vi "CRYGet Heterodyne Curve.vi"(9 "Unit Info In":T5={"Y unit In"="dB", "dB ref In"=1.0, "Y unit Out"="dB", "dB ref Out"=1.0, "Y unit Curve"="dB", "dB ref Curve"=1.0, "Y data  Curve"=0, "Y data Time"=0}, 10 "Additive Info":T3, 11 "Impedance and Mic Current In":bool[](array[boolean])) -> (1 "Display Array":T4(array[cluster]), 2 "Unit Info Out":T2[](array[typedef]), 3 "Curve Info Array Out":T1)   [LabVIEW 2013]
uses:
  Typedef Control/CRYUnit Info Cluster.ctl
  Typedef Control/CRYUnit Info Out Cluster.ctl
  Typedef Control/CRYAnalysis CurveName Cluster.ctl
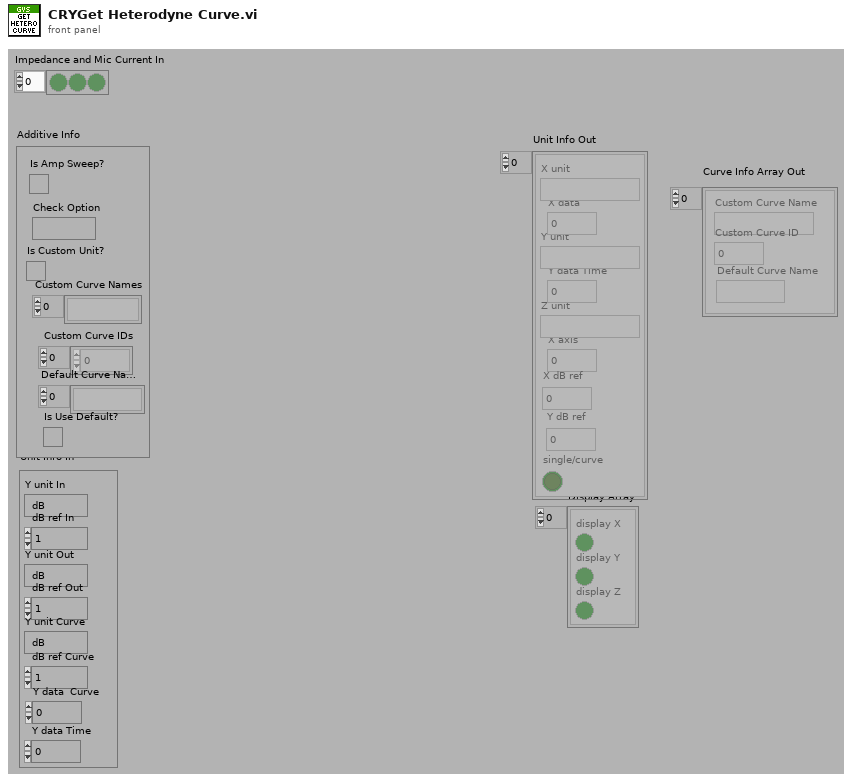
[diagram p1: front panel]
types:
  T1 = typedef "CRYAnalysis CurveName Cluster.ctl" = cluster{"Custom Curve Name":string, "Custom Curve ID":i32, "Default Curve Name":string}[]
  T2 = typedef "CRYUnit Info Out Cluster.ctl" = cluster{"X unit":string, "X data":u16, "Y unit":string, "Y data Time":u16, "Z unit":string, "X axis":u16, "X dB ref":dbl, "Y dB ref":dbl, "single/curve":bool}
  T3 = cluster{"Is Amp Sweep?":bool, "Check Option":string, "Is Custom Unit?":bool, "Custom Curve Names":string[], "Custom Curve IDs":i32[], "Default Curve Names":string[], "Is Use Default?":bool}
  T4 = cluster{"display X":bool, "display Y":bool, "display Z":bool}[]
  T5 = typedef "CRYUnit Info Cluster.ctl" = cluster{"Y unit In":string, "dB ref In":dbl, "Y unit Out":string, "dB ref Out":dbl, "Y unit Curve":string, "dB ref Curve":dbl, "Y data  Curve":u16, "Y data Time":u16}
  T6 = cluster{"display X":bool, "display Y":bool, "display Z":bool}
  T7 = enum32{"English", "Chinese", "Korean", "Japanese", "Russian", "Chinese traditional"}
  T8 = cluster{"Y unit Out":string, "dB":u16, "Y unit Curve":string, "Y data  Curve":u16, "Y unit Curve":string, "Lin":u16, "dB ref Out":dbl, "dB ref Curve":dbl, "display X":bool}
  T9 = cluster{"Y unit Out":string, "dB":u16, "Y unit Curve":string, "Y data  Curve":u16, "Y unit Curve":string, "Lin":u16, "dB ref Out":dbl, "dB ref Curve":dbl, "display X":bool}[]
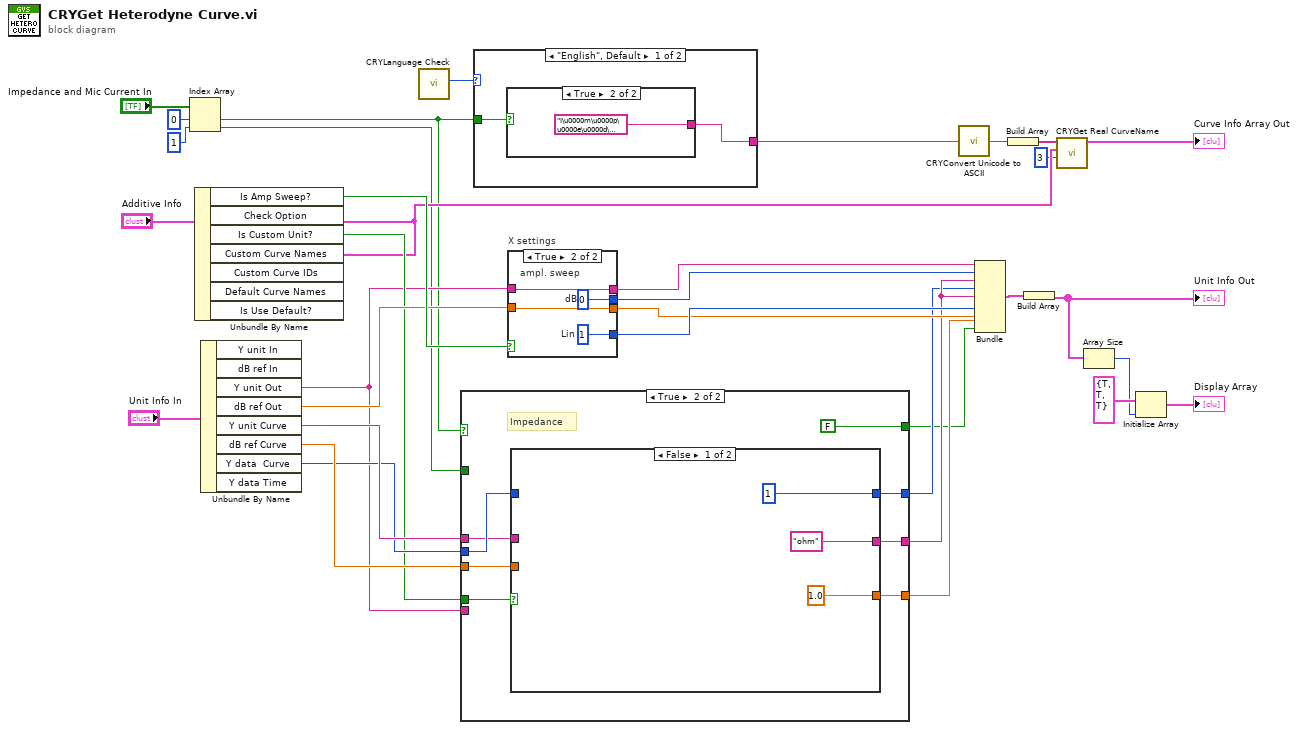
[diagram p0: block diagram]
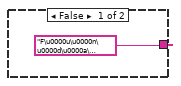
[diagram p2: hidden frame]
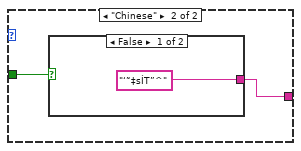
[diagram p3: hidden frame]
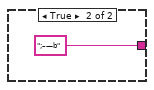
[diagram p4: hidden frame]
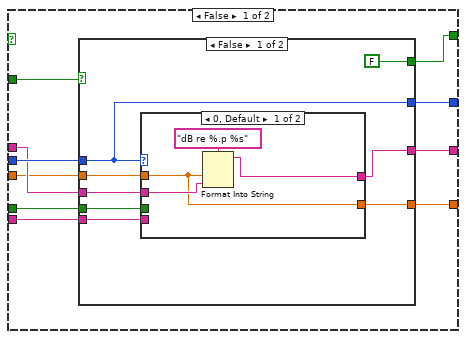
[diagram p5: hidden frame]
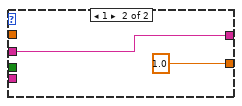
[diagram p6: hidden frame]
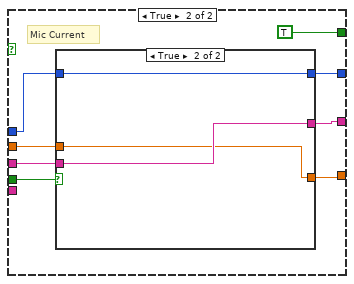
[diagram p7: hidden frame]
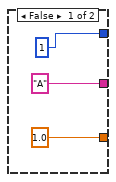
[diagram p8: hidden frame]
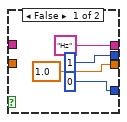
[diagram p10: hidden frame]
diagram:
  n1 = Index Array(array="Impedance and Mic Current In", index #1=0 ("index"), index #2=1 ("index")) -> (element #1=w4:bool, element #2=w3:bool)
  n2 = Unbundle By Name("Additive Info") -> ("Is Amp Sweep?"=w30:bool, "Is Custom Unit?"=w16:bool)  [unwired: 5 out]
  n3 = Unbundle By Name("Unit Info In") -> ("Y unit Out"=w15:string, "dB ref Out"=w29:dbl, "Y unit Curve"=w20:string, "dB ref Curve"=w21:dbl, "Y data  Curve"=w17:u16)  [unwired: 3 out]
  n4 = call "CRYLanguage Check.vi"() -> ("Language"=w8:T7)  [unwired: 10 in, 1 out]
  n5 = case shown="True" w4 {
    tunnel: w20 -> [w41 w74]
    tunnel: [w42 w79] -> w19
    tunnel: w17 -> [w43 w76]
    tunnel: w21 -> [w40 w73]
    tunnel: [w39 w78] -> w18
    tunnel: w16 -> [w38 w77]
    tunnel: w15 -> [w37 _]
    tunnel: w3 -> [w36 _]
    tunnel: [w35 w75] -> w2
    tunnel: [w34 FALSE ("display X")] -> w1
    frame False {
      n6 = case shown="False" w36 {
        tunnel: w43 -> [w45 w61]
        tunnel: [w51 w63] -> w42
        tunnel: w41 -> [w50 w60]
        tunnel: w40 -> [w49 w59]
        tunnel: [w48 w62] -> w39
        tunnel: w38 -> [w47 w65]
        tunnel: w37 -> [w46 _]
        tunnel: [w45 w64] -> w35
        tunnel: [FALSE ("display X") TRUE ("display X")] -> w34
        frame False {
          n7 = case shown="0, Default" w45 {
            tunnel: [w52 w56] -> w51
            tunnel: w49 -> [w53 _]
            tunnel: w50 -> [w54 w56]
            tunnel: [w53 1.0 ("dB ref Curve")] -> w48
            tunnel: w47 -> [_ _]
            tunnel: w46 -> [_ _]
            frame 0, Default {
              n8 = Format Into String(format string="dB re %.p %s", w53, w54) -> (resulting string=w52:string)  [unwired: 2 in, 1 out]
            }
            frame 1 {
            }
          }
        }
        frame True {
          # "Mic Current"
          n9 = case shown="True" w65 {
            tunnel: [u16 1 ("Y data  Curve") w71] -> w64
            tunnel: ["A" ("unit") w70] -> w63
            tunnel: [1.0 ("dB ref Curve") w69] -> w62
            tunnel: w61 -> [_ w71]
            tunnel: w60 -> [_ w70]
            tunnel: w59 -> [_ w69]
            frame False {
            }
            frame True {
            }
          }
        }
      }
    }
    frame True {
      # "Impedance"
      n10 = case shown="False" w77 {
        tunnel: ["ohm" ("unit") w84] -> w79
        tunnel: [1.0 ("dB ref Curve") w83] -> w78
        tunnel: w76 -> [_ w85]
        tunnel: [u16 1 ("Y data  Curve") w85] -> w75
        tunnel: w74 -> [_ w84]
        tunnel: w73 -> [_ w83]
        frame False {
        }
        frame True {
        }
      }
    }
  }
  n11 = case shown="\"English\", Default" w8 {
    tunnel: w4 -> [w87 w91]
    tunnel: [w86 w90] -> w10
    frame "English", Default {
      n12 = case shown="True" w87 {
        tunnel: ["F\u0000u\u0000n\u0000d\u0000a\u0000m\u0000e\u0000n\u0000t\u0000a\u0000l\u0000" ("Label.Text") "I\u0000m\u0000p\u0000e\u0000d\u0000a\u0000n\u0000c\u0000e\u0000" ("Label.Text")] -> w86
        frame False {
        }
        frame True {
        }
      }
    }
    frame "Chinese" {
      n13 = case shown="False" w91 {
        tunnel: ["‘˜‡sÍT”^" ("Label.Text") ";–—b" ("Label.Text")] -> w90
        frame False {
        }
        frame True {
        }
      }
    }
  }
  n14 = case "X settings" shown="True" w30 {
    tunnel: ["Hz" ("X unit") w99] -> w28
    tunnel: [u16 1 ("Y data") w100] -> w27
    tunnel: [1.0 ("X dB ref") w98] -> w25
    tunnel: [u16 0 ("X axis") w101] -> w26
    tunnel: w15 -> [_ w99]
    tunnel: w29 -> [_ w98]
    frame False {
    }
    frame True {
      w100 = u16 0  # dB
      w101 = u16 1  # Lin
      # "ampl. sweep"
    }
  }
  n15 = call "CRYConvert Unicode to ASCII.vi"("Unicode"=w10) -> ("ASCII"=w11:string)  [unwired: 4 in]
  n16 = Bundle("Y unit Out"=w28, "dB"=w27, "Y unit Curve"=w19, "Y data  Curve"=w2, "Y unit Curve"=w19, "Lin"=w26, "dB ref Out"=w25, "dB ref Curve"=w18, "display X"=w1) -> (w23:T8)  [unwired: 1 in]
  n17 = Build Array(w11) -> (w9:string[])
  n18 = Build Array(w23) -> (w22:T9)
  "Unit Info Out" <- w22
  n19 = call "CRYGet Real CurveName.vi"("Key No"=3, "Additive Info"="Additive Info", "CurveArrayByType"=w9) -> ("Curve Info Array Out"=→"Curve Info Array Out":T1)  [unwired: 8 in]
  n20 = Array Size(array=w22) -> (size(s)=w32:i32)
  n21 = Initialize Array(T6 {"display X"=TRUE, "display Y"=TRUE, "display Z"=TRUE}, w32) -> (→"Display Array":T4)
